vi "CIS.vi"(2 "Run uninterrupted?":bool, 3 "Device Category IN:":string(combo)="ATLAS18SS" caption="Device Category:", 4 "Structure:":string, 5 "Sensor Serial No.:":string, 6 "DB Serial No.:":string) -> (0 "Done!":bool)   [LabVIEW 2019]
doc: "Performs Cis measurements according to ATLAS ITk Quality Control Specifications."
uses:
  general_VIs/globals/QC_MeasurementSetup.vi
  general_VIs/globals/QC_RunInformation.vi
  InstrControl/InstrumentSetup.vi
  InstrControl/Switching/Switching.lvclass
  InstrControl/SupplyControl/SupplyControl.lvclass
  InstrControl/LCRControl/LCRControl.lvclass
  InstrControl/ArduinoControl/ArduinoControl.lvclass
  <vilib>/Analysis/NI_AALBase.lvlib
  InstrControl/InstrControl.lvclass
panel:
  out "Tab Control 2":enum32{"Cis Setup", "Cis Scan"}(tab)
  in  "Current Limit [µA]":dbl=1000.0 min=0.0001 format="%.3f"
  in  "Cis @300V limit [pF/cm]":dbl=1.0
  in  "step interval [s] IN":i32=5 caption="step interval [s]"
  in  "step [V] IN":dbl=10.0 caption="step [V]" format="%.1f"
  in  "Final volts [V] IN":dbl=-500.0 caption="Final volts [V]"
  in  "Initial volts [V] IN":dbl caption="Initial volts [V]"
  in  "Frequency [Hz] Setup":i32=500 caption="Frequency [Hz]" format="%#.3p"
  in  "Measurement Configurations":bool
  in  "Continue":bool
  in  "Quit":bool
  in  "Software current limit?":bool
  out "Capacitance":dbl[](array[numeric]) caption="Cap [pF]"
  out "Volts":dbl[](array[numeric]) caption="Volts [V]"
  out "Resistance":dbl[](array[numeric]) caption="Res [kOhm]"
  out "step interval [s]":u32=5
  out "step [V]":dbl=10.0 format="%.1f"
  out "Final volts [V]":dbl=-700.0 format="%.1f"
  out "Initial volts [V]":dbl format="%.1f"
  out "Frequency [Hz]":i32=100000 format="%#.3p"
  out "RH":dbl[](array[numeric]) caption="RH [%]" format="%#.2f"
  out "Temp.":dbl[](array[numeric]) caption="Temp. [°C]" format="%#.2f"
  out "Cgraph":cluster{"Initial volts":dbl, dbl, dbl[]}(graph)
  in  "Scales":T1(ring)
  in  "Cscale":enum16{"1/C^2 [1/nF^2]", "nF", "pF"}(ring)=enum."pF"
  out "positive ramp?":bool
  out "Tab Control":enum32{"Cis Setup", "Cis Scan"}(tab)
  in  "Switching":string(combo)="Pickering Matrix"
  in  "LCR Meter":string(combo)="WayneKerr 6440B"
  in  "Cis Supply":string(combo)="Keithley 2410"
  in  "Temperature":enum16{"Read Arduino", "Enter manually"}(ring)
  in  "User:":string(combo)="Christoph"
  in  "Manufacturer:":string(combo)="Hamamatsu"
  in  "abort":bool
  out "Device Category:":string
  out "DB Serial No.:":string
  out "Current Volts:":dbl format="%.2f"
  in  "quit (no save)":bool
  in  "Quit & Save":bool
  out "Bias On/Off:":bool
  out "STATUS 1":string
  out "Initiated:":string
  out "Sensor No.:":string
  out "No of steps":u32
  out "Current reading No.":u32
  out "Last reading at:":string
  # "University of\nCambridge"
  # "Strip Sensor QC: inter-strip Capacitance"
  # "Vertical Scale:"
  # "Measurement Configuration"
  # "Cis Scan parameters:"
  # "Last 5 readings:"
  # "n-4"
  # "n-3"
  # "n-2"
  # "n-1"
  # "n"
  # "DUT Description"
  # "Hardware"
  # "DUT & Test Description:"
  # "Current status:"
  # "Rdg No:"
  # "out of"
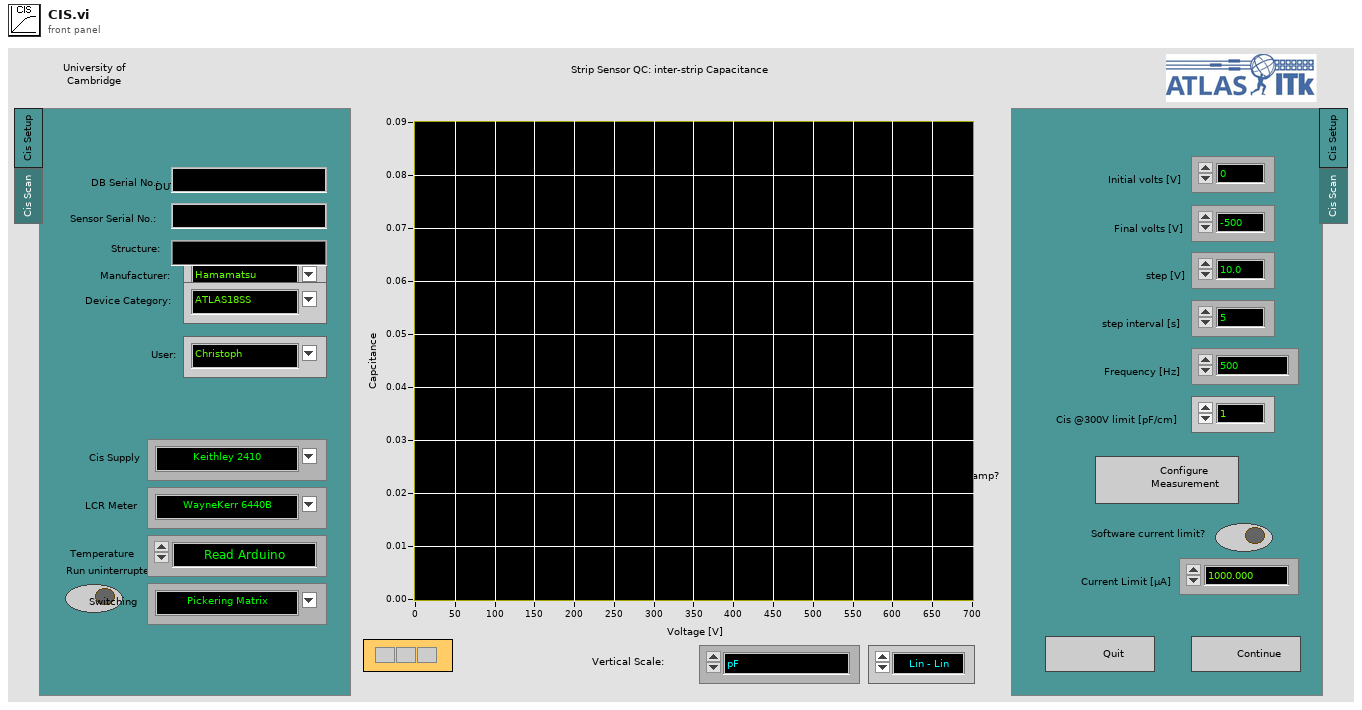
[diagram p1: front panel]
types:
  T1 = enum16{"Lin - Lin", "Log - Lin", "Lin - Log", "Log - log"}
  T2 = enum16{"Supply", "LCR", "Multimeter", "Switching"}
  T3 = enum16{"Reset", "Read Array", "Read Element", "Write Element", "Write Array", "Add Element", "Add Array"}
  T4 = enum16{"Reset", "Ground", "Striptest Bias", "Striptest SMU", "Striptest LCR", "IV", "CV", "Interstrip Cap", "Interstrip Res"}
  T5 = enum32{"IV", "CV", "Stability", "Striptest", "Cis", "Ris", "PTP"}
  T6 = cluster{"Sensor Serial No.:":string, "Wafer Serial No.:":string, "Batch:":string, "Manufacturer:":string, "Device Category:":string, "Database Serial No.:":string, "Date Initiated:":string, "Time Initiated:":string, "Test":string, "Instruments used:":string, "Probeplan used:":string, "End of Run comment:":string, "User:":string}
  T7 = cluster{"Institute":string, "Manufacturers":string[], "Devices":string[], "Serialnumbers Lookup DB":string, "Data directory":string, "Backup & screenshot directory":string, "List of known users":string[], "Measurement switch not used":bool, "Measurement Switch":string, "DUT Switch":string}
  T8 = cluster{"Supply":refnum<class "SupplyControl.lvclass">, "LCR":refnum<class "LCRControl.lvclass">, "Initial Voltage [V]":dbl, "Final Voltage [V]":dbl, "Step Size [V]":dbl, "Step Interval [s]":i32, "Number Of Steps":u32, "AC frequency [Hz]":i32, "RC Configuration":u16, "AC amplitude [V]":dbl, "Ramp down steps [V]":dbl, "Ramp down Interval [s]":i32, "Set Current Limit?":bool, "Current Limit [µA]":dbl, "Temperature Readout":enum16{"Read Arduino", "Enter manually"}, "Arduino":refnum<class "ArduinoControl.lvclass">, "Supply Name":string, "LCR Name":string, "C_is Limit [pF/cm]":dbl, "Switching":refnum<class "Switching.lvclass">, "Matrix used?":bool, "Matrix X Channels":cluster{"Bias Supply / SMU LO":i32, "Bias Supply / SMU HI":i32, "CV Box LO":i32, "CV Box HI":i32, "CV Box LO IN":i32, "CV Box HI IN":i32, "Volt meter LO":i32, "Volt meter HI":i32, "Mux1 C1":i32, "Mux1 C2":i32, "Mux2 C1":i32, "Mux2 C2":i32}, "Structure Name":string}
  T9 = cluster{"VISA address":refnum<visa-resource-name>, "T sensor":enum16{"SHT", "DS"}, "Arduino":refnum<class "ArduinoControl.lvclass">}
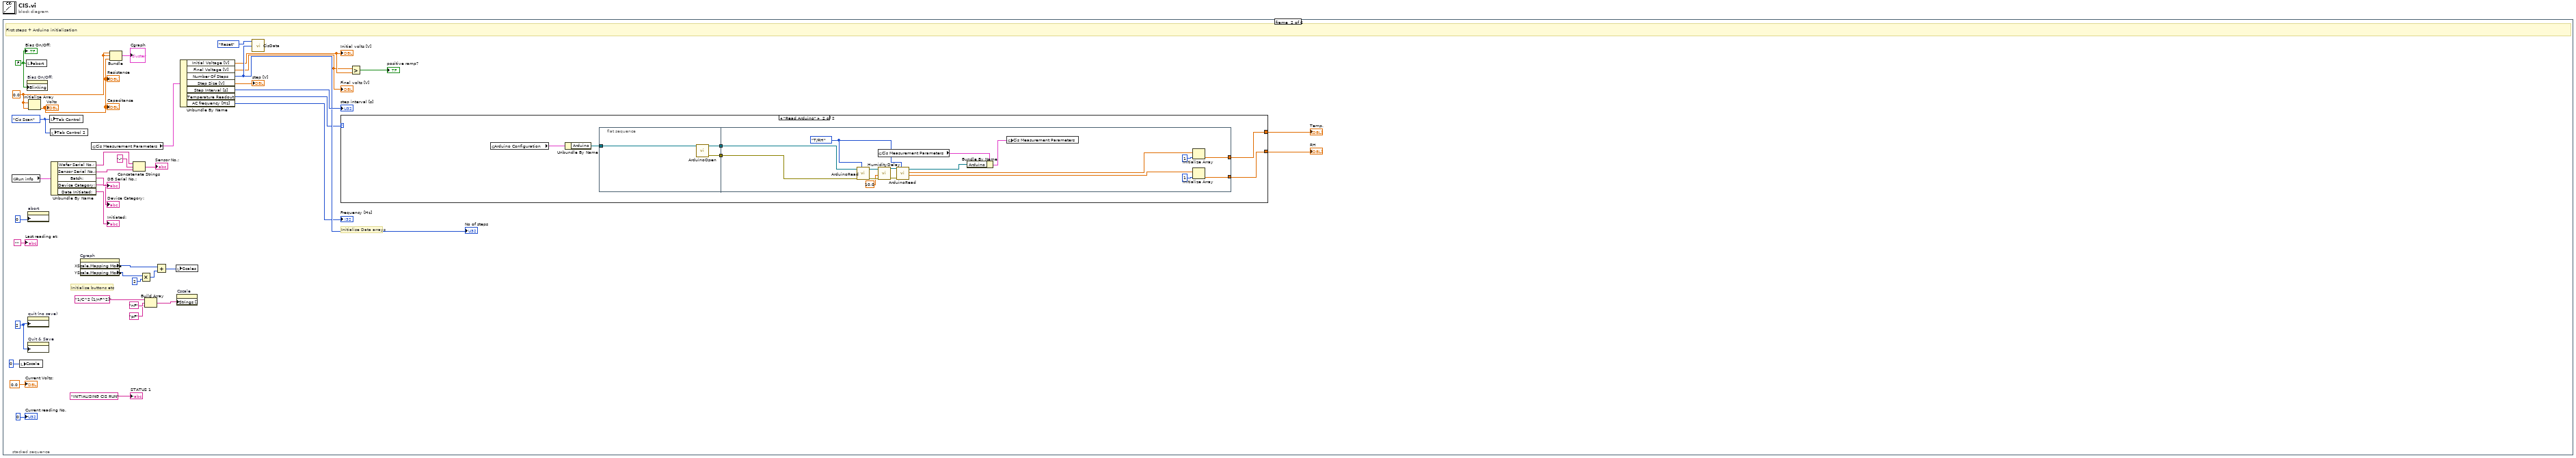
[diagram p0: block diagram]
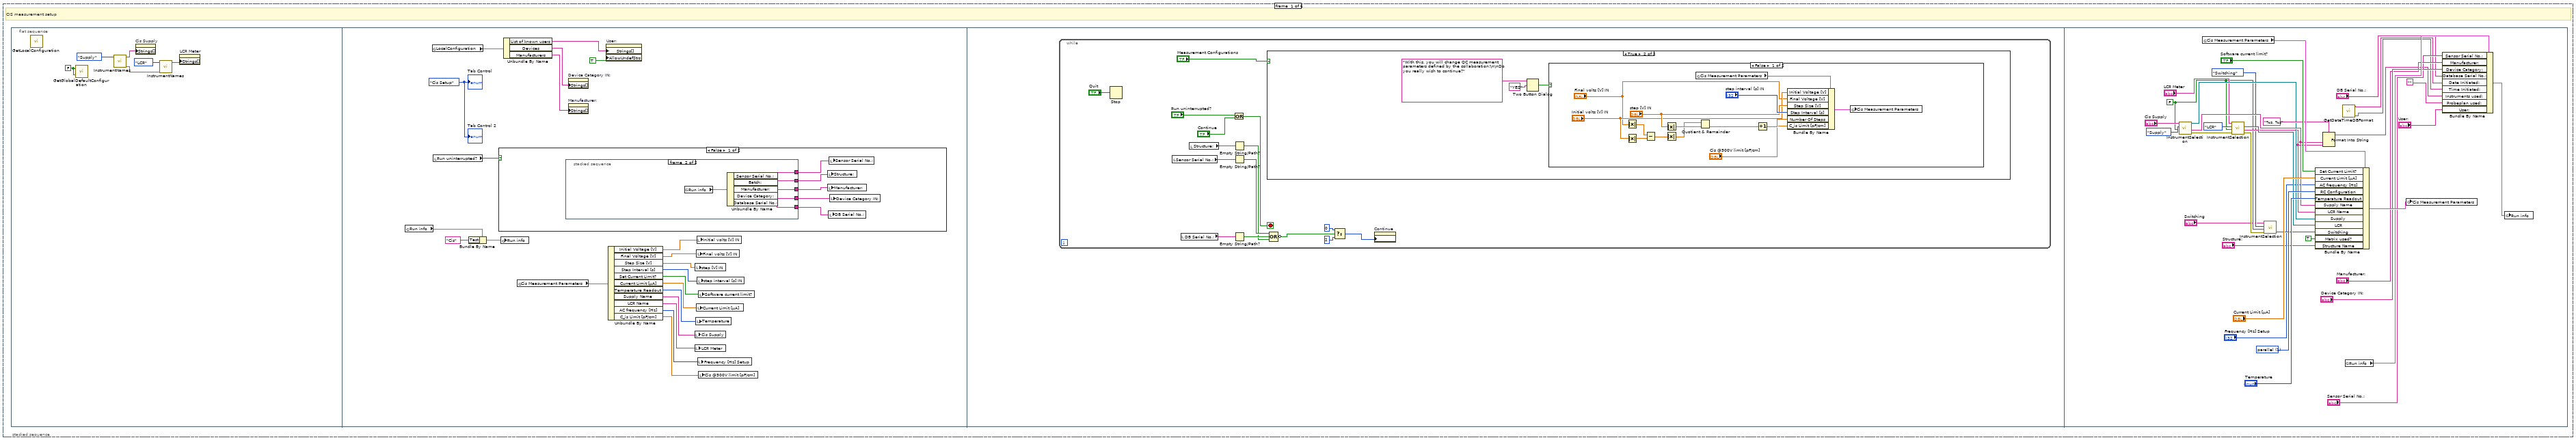
[diagram p2: hidden frame]
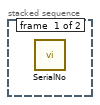
[diagram p3: hidden frame]
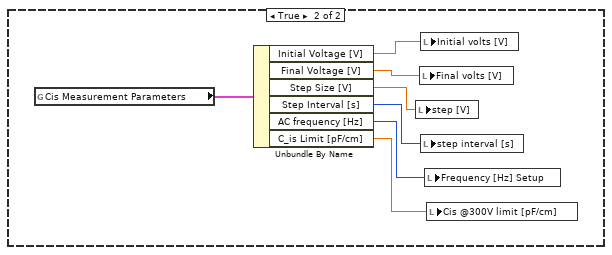
[diagram p6: hidden frame]
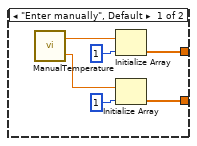
[diagram p7: hidden frame]
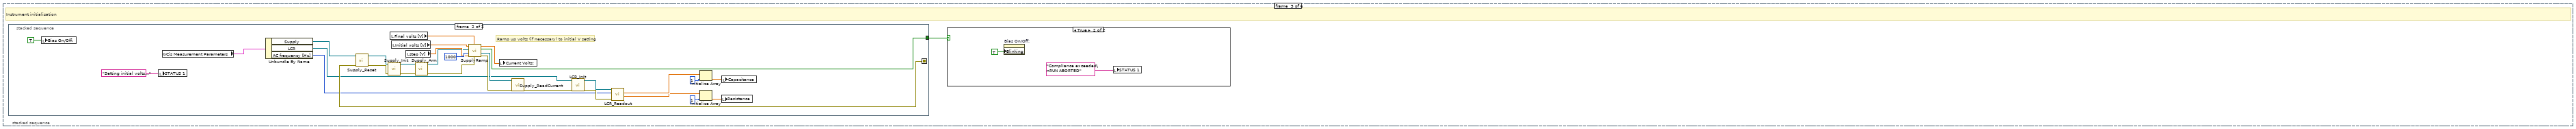
[diagram p8: hidden frame]
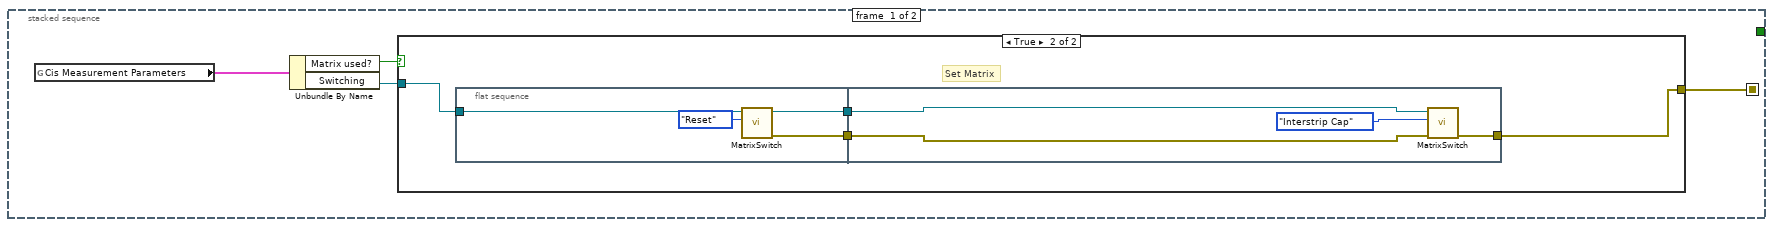
[diagram p9: hidden frame]
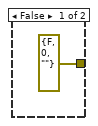
[diagram p10: hidden frame]
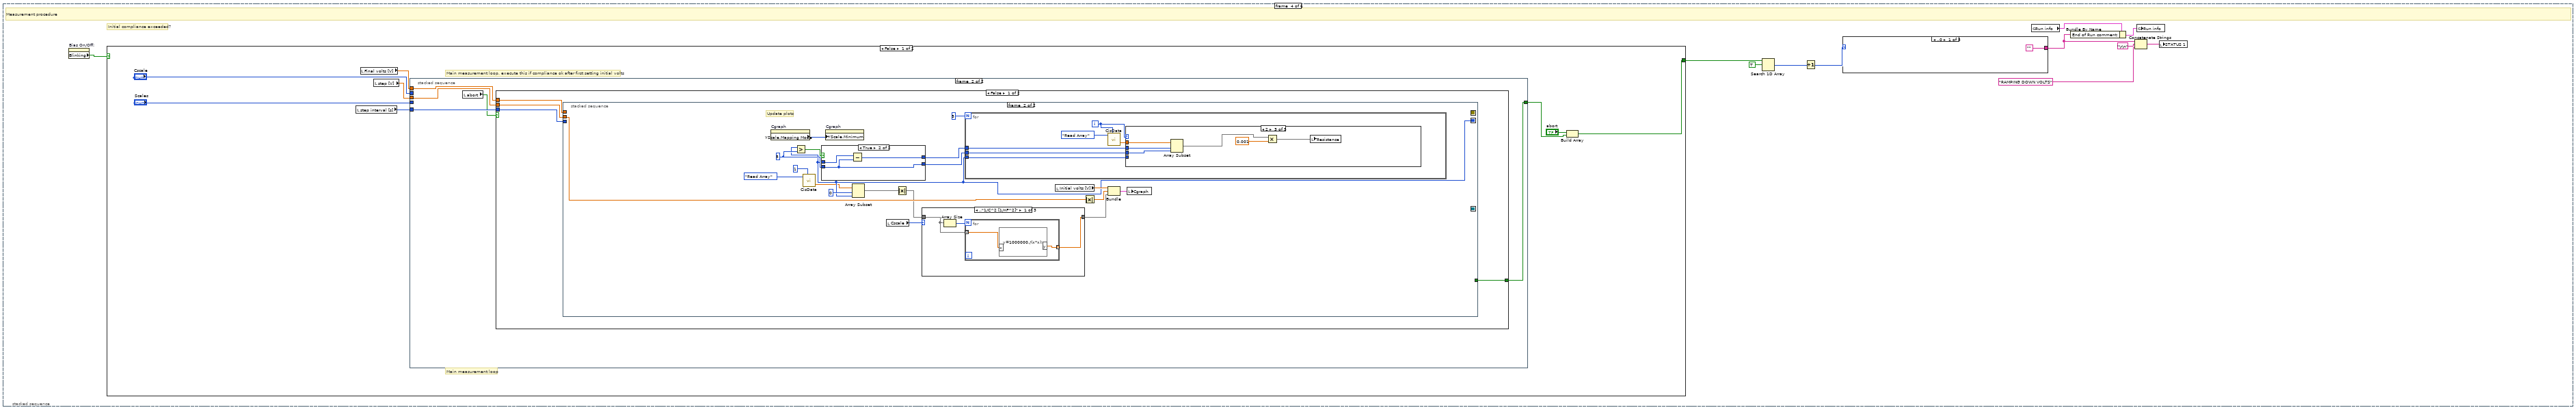
[diagram p12: hidden frame]
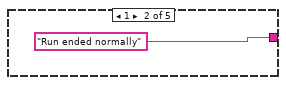
[diagram p13: hidden frame]
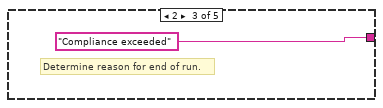
[diagram p14: hidden frame]
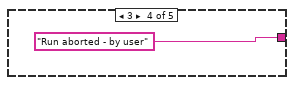
[diagram p15: hidden frame]
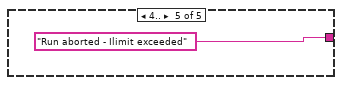
[diagram p16: hidden frame]
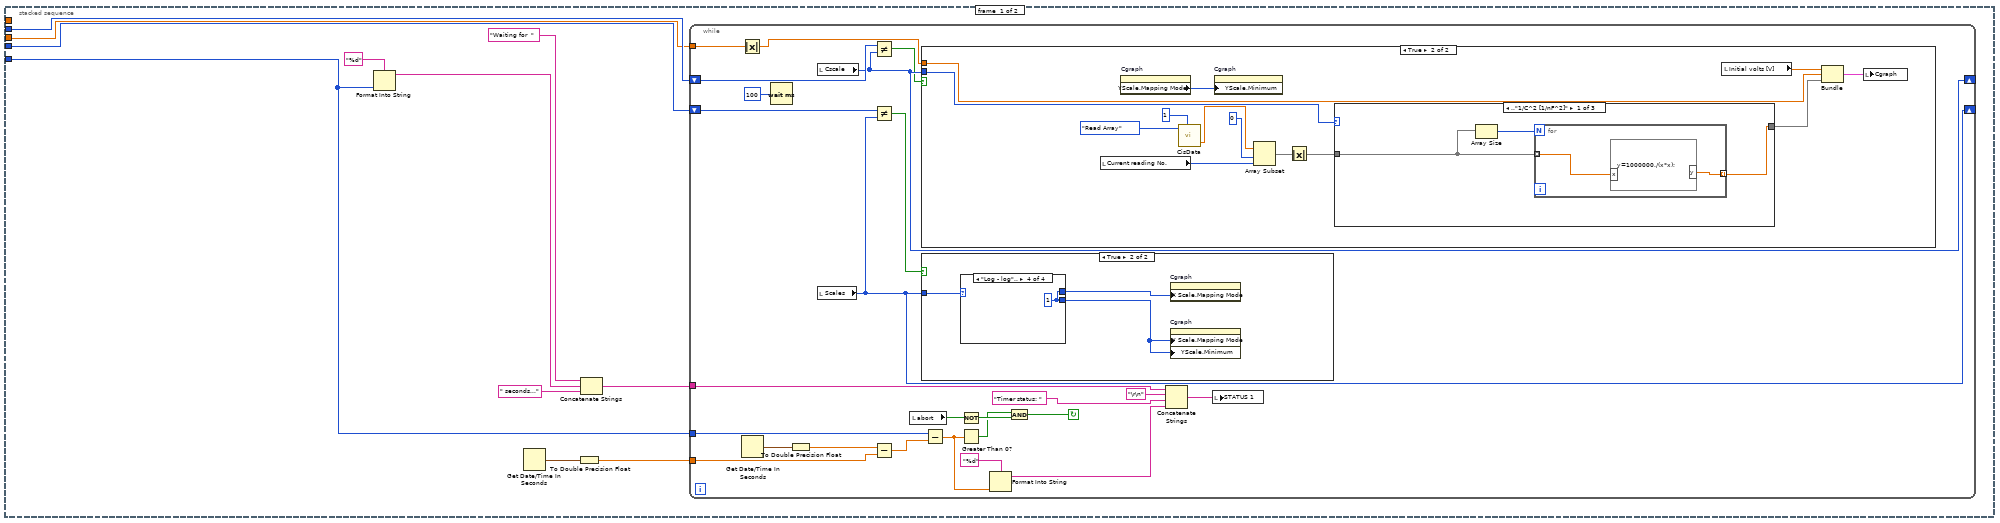
[diagram p17: hidden frame]
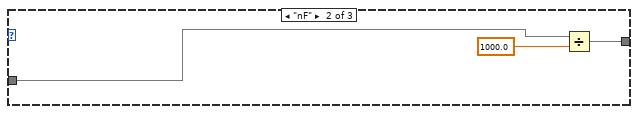
[diagram p19: hidden frame]
diagram:
  n1 = stacked-sequence {
    frame #0 {
      # "CIS measurement setup"
      n2 = flat-sequence {
        frame #0 {
          w6 = FALSE
          n3 = call "GetLocalConfiguration.vi"() -> ()  [unwired: 3 in, 1 out]
          n4 = call "GetGlobalDefaultConfiguration.vi"("DO NOT override instruments"=w6, "Read defaults?"=w6) -> ()  [unwired: 1 in, 1 out]
          n5 = call "InstrumentNames.vi"("Instrument type"=T2."Supply") -> ("error out"=w3:errorcluster, "Instrument names"=w1:string[])  [unwired: 9 in]
          n6 = property on="Cis Supply" class="CmbBox"("Strings[]"=w1) -> ()  [unwired: 2 in, 2 out]
          n7 = call "InstrumentNames.vi"("error in (no error)"=w3, "Instrument type"=T2."LCR") -> ("Instrument names"=w2:string[])  [unwired: 8 in, 1 out]
          n8 = property on="LCR Meter" class="CmbBox"("Strings[]"=w2) -> ()  [unwired: 2 in, 2 out]
        }
        frame #1 {
          w15 = enum32{"Cis Setup", "Cis Scan"}."Cis Setup" ("Tab Control")
          n9 = global read "QC_RunInformation.vi" "Run info"() -> (w16:T6)
          n10 = global read "QC_RunInformation.vi" "LocalConfiguration"() -> (w23:T7)
          n11 = local read "Run uninterrupted?"() -> (w14:bool)
          n12 = Bundle By Name(cluster=w16, "Test"="Cis") -> (w18:T6)
          n13 = case shown="False" w14 {
            frame False {
              n14 = stacked-sequence {
                tunnel: [_ w39] -> w33
                tunnel: [_ w38] -> w32
                tunnel: [_ w37] -> w31
                tunnel: [_ w36] -> w29
                tunnel: [_ w34] -> w30
                frame #0 {
                  n15 = call "SerialNo.vi"() -> ()  [unwired: 5 in, 1 out]
                }
                frame #1 {
                  n16 = global read "QC_RunInformation.vi" "Run info"() -> (w35:T6)
                  n17 = Unbundle By Name(w35) -> ("Sensor Serial No.:"=w39:string, "Batch:"=w38:string, "Manufacturer:"=w37:string, "Device Category:"=w36:string, "Database Serial No.:"=w34:string)
                }
              }
              n18 = local write "Structure:"(w32) -> ()
              n19 = local write "Manufacturer:"(w31) -> ()
              n20 = local write "DB Serial No.:"(w30) -> ()
              n21 = local write "Sensor Serial No.:"(w33) -> ()
              n22 = local write "Device Category IN:"(w29) -> ()
            }
            frame True {
            }
          }
          n23 = global write "QC_RunInformation.vi" "Run info"(w18) -> ()
          n24 = Unbundle By Name(w23) -> ("List of known users"=w22:string[], "Devices"=w7:string[], "Manufacturers"=w8:string[])
          n25 = global read "QC_MeasurementSetup.vi" "Cis Measurement Parameters"() -> (w26:T8)
          n26 = property on="Device Category IN:" class="CmbBox"("Strings[]"=w7) -> ()  [unwired: 2 in, 2 out]
          n27 = property on="Manufacturer:" class="CmbBox"("Strings[]"=w8) -> ()  [unwired: 2 in, 2 out]
          n28 = property on="User:" class="CmbBox"("Strings[]"=w22, "AllowUndefStrs"=TRUE) -> ()  [unwired: 2 in, 2 out]
          n29 = Unbundle By Name(w26) -> ("Initial Voltage [V]"=w11:dbl, "Final Voltage [V]"=w12:dbl, "Step Size [V]"=w10:dbl, "Step Interval [s]"=w13:i32, "Set Current Limit?"=w25:bool, "Current Limit [µA]"=w24:dbl, "Temperature Readout"=w28:enum16{"Read Arduino", "Enter manually"}, "Supply Name"=w27:string, "LCR Name"=w20:string, "AC frequency [Hz]"=w19:i32, "C_is Limit [pF/cm]"=w9:dbl)
          n30 = local write "Cis Supply"(w27) -> ()
          n31 = local write "LCR Meter"(w20) -> ()
          n32 = local write "step [V] IN"(w10) -> ()
          n33 = local write "Temperature"(w28) -> ()
          n34 = local write "Final volts [V] IN"(w12) -> ()
          n35 = local write "Current Limit [µA]"(w24) -> ()
          n36 = local write "Initial volts [V] IN"(w11) -> ()
          n37 = local write "step interval [s] IN"(w13) -> ()
          n38 = local write "Frequency [Hz] Setup"(w19) -> ()
          n39 = local write "Software current limit?"(w25) -> ()
          n40 = local write "Cis @300V limit [pF/cm]"(w9) -> ()
          "Tab Control" <- w15
          "Tab Control 2" <- w15
        }
        frame #2 {
          n41 = while {
            stop <- w41 stop-if-true
            n42 = Stop(stop? (T)="Quit") -> ()
            n43 = local read "Sensor Serial No.:"() -> (w53:string)
            n44 = local read "DB Serial No.:"() -> (w52:string)
            n45 = local read "Structure:"() -> (w45:string)
            n46 = Or(x="Run uninterrupted?", y="Continue") -> (x .or. y?=w41:bool)
            n47 = Empty String/Path?(string/path=w45) -> (empty?=w44:bool)
            n48 = Empty String/Path?(string/path=w53) -> (empty?=w50:bool)
            n49 = Empty String/Path?(string/path=w52) -> (empty?=w51:bool)
            n50 = case shown="True" "Measurement Configurations" {
              frame False {
              }
              frame True {
                n51 = Two Button Dialog(message="With this, you will change QC measurement parameters defined by the collaboration!\n\nDo you really wish to continue?", 2:"YES") -> (T button?=w55:bool)  [unwired: 1 in]
                n52 = case shown="False" w55 {
                  frame False {
                    n53 = Absolute Value(x="Final volts [V] IN") -> (abs(x)=w68:dbl)
                    n54 = Absolute Value(x="Initial volts [V] IN") -> (abs(x)=w67:dbl)
                    n55 = Subtract(x=w68, y=w67) -> (x-y=w65:dbl)
                    n56 = Absolute Value(x="step [V] IN") -> (abs(x)=w66:dbl)
                    n57 = Absolute Value(x=w65) -> (abs(x)=w61:dbl)
                    n58 = global read "QC_MeasurementSetup.vi" "Cis Measurement Parameters"() -> (w70:T8)
                    n59 = Quotient & Remainder(x=w61, y=w66) -> (floor(x/y)=w69:dbl)  [unwired: 1 out]
                    n60 = Increment(x=w69) -> (x+1=w64:dbl)
                    n61 = Bundle By Name(cluster=w70, "Initial Voltage [V]"="Initial volts [V] IN", "Final Voltage [V]"="Final volts [V] IN", "Step Size [V]"="step [V] IN", "Step Interval [s]"="step interval [s] IN", "Number Of Steps"=w64, "C_is Limit [pF/cm]"="Cis @300V limit [pF/cm]") -> (w71:T8)
                    n62 = global write "QC_MeasurementSetup.vi" "Cis Measurement Parameters"(w71) -> ()
                  }
                  frame True {
                    n63 = global read "QC_MeasurementSetup.vi" "Cis Measurement Parameters"() -> (w78:T8)
                    n64 = Unbundle By Name(w78) -> ("Initial Voltage [V]"=w76:dbl, "Final Voltage [V]"=w77:dbl, "Step Size [V]"=w75:dbl, "Step Interval [s]"=w74:i32, "AC frequency [Hz]"=w73:i32, "C_is Limit [pF/cm]"=w72:dbl)
                    n65 = local write "step [V]"(w75) -> ()
                    n66 = local write "Final volts [V]"(w77) -> ()
                    n67 = local write "Initial volts [V]"(w76) -> ()
                    n68 = local write "step interval [s]"(w74) -> ()
                    n69 = local write "Frequency [Hz] Setup"(w73) -> ()
                    n70 = local write "Cis @300V limit [pF/cm]"(w72) -> ()
                  }
                }
              }
            }
            n71 = Compound Arithmetic op=OR(w50, w51, w44) -> (invert w49:bool)
            n72 = Select(t=0, s=w49, f=2) -> (s? t:f=w46:i32)
            n73 = property on="Continue" class="Bool"("DisabledEnum"=w46) -> ()  [unwired: 2 in, 2 out]
          }
        }
        frame #3 {
          w87 = FALSE
          w102 = u16 1 items=["serial", "parallel"] ("RC Configuration")
          n74 = call "InstrumentSelection.vi"("Verify GPIB address"=w87, "Instrument type"=T2."Supply", "Instrument name IN"="Cis Supply") -> ("error out"=w92:errorcluster, "Instrument name OUT"=w97:string, "Supply"=w96:refnum<class "SupplyControl.lvclass">)  [unwired: 3 in, 3 out]
          n75 = global read "QC_MeasurementSetup.vi" "Cis Measurement Parameters"() -> (w112:T8)
          n76 = call "InstrumentSelection.vi"("error in (no error)"=w92, "Verify GPIB address"=w87, "Instrument type"=T2."LCR", "Instrument name IN"="LCR Meter") -> ("error out"=w88:errorcluster, "Instrument name OUT"=w93:string, "LCR"=w95:refnum<class "LCRControl.lvclass">)  [unwired: 2 in, 3 out]
          n77 = call "InstrumentSelection.vi"("error in (no error)"=w88, "Verify GPIB address"=w87, "Instrument type"=T2."Switching", "Instrument name IN"="Switching") -> ("Switching"=w86:refnum<class "Switching.lvclass">)  [unwired: 2 in, 5 out]
          n78 = Bundle By Name(cluster=w112, "Set Current Limit?"="Software current limit?", "Current Limit [µA]"="Current Limit [µA]", "AC frequency [Hz]"="Frequency [Hz] Setup", "RC Configuration"=w102, "Temperature Readout"="Temperature", "Supply Name"=w97, "LCR Name"=w93, "Supply"=w96, "LCR"=w95, "Switching"=w86, "Matrix used?"=TRUE, "Structure Name"="Structure:") -> (w113:T8)
          n79 = Format Into String(format string="%s, %s", w97, w93) -> (resulting string=w99:string)  [unwired: 2 in, 1 out]
          n80 = call "GetDateTimeDBFormat.vi"() -> ("Time in 24h format, e.g. 13:40:54"=w79:string, "Abbreviated Date, e.g. 13 Nov 2020"=w80:string)  [unwired: 10 in]
          n81 = global read "QC_RunInformation.vi" "Run info"() -> (w109:T6)
          n82 = global write "QC_MeasurementSetup.vi" "Cis Measurement Parameters"(w113) -> ()
          n83 = Bundle By Name(cluster=w109, "Sensor Serial No.:"="Sensor Serial No.:", "Manufacturer:"="Manufacturer:", "Device Category:"="Device Category IN:", "Database Serial No.:"="DB Serial No.:", "Date Initiated:"=w80, "Time Initiated:"=w79, "Instruments used:"=w99, "Probeplan used:"="", "User:"="User:") -> (w108:T6)
          n84 = global write "QC_RunInformation.vi" "Run info"(w108) -> ()
        }
      }
    }
    frame #1 {
      w114 = enum32{"Cis Setup", "Cis Scan"}."Cis Scan" ("Tab Control")
      w136 = 2
      w143 = 0.0
      w135 = FALSE ("Visible")
      # "Initialise buttons etc"
      # "Initialise Data arrays"
      # "First steps + Arduino initialisation"
      n85 = global read "QC_RunInformation.vi" "Run info"() -> (w153:T6)
      n86 = local write "Cscale"(u16 0 ("Scale")) -> ()
      n87 = local write "abort"(w135) -> ()
      n88 = property on="Bias On/Off:" class="Bool (strict)"("Blinking"=w135) -> ()  [unwired: 2 in, 2 out]
      n89 = property on="abort" class="Bool (strict)"("DisabledEnum"=0) -> ()  [unwired: 2 in, 2 out]
      n90 = property on="quit (no save)" class="Bool"("DisabledEnum"=w136) -> ()  [unwired: 2 in, 2 out]
      n91 = property on="Quit & Save" class="Bool"("DisabledEnum"=w136) -> ()  [unwired: 2 in, 2 out]
      n92 = Initialize Array(w143, w143) -> (w116:dbl[])
      "Volts" <- w116
      "Capacitance" <- w116
      "Resistance" <- w116
      n93 = local write "Tab Control"(w114) -> ()
      n94 = local write "Tab Control 2"(w114) -> ()
      n95 = Unbundle By Name(w153) -> ("Wafer Serial No.:"=w122:string, "Sensor Serial No.:"=w121:string, "Batch:"=→"DB Serial No.:":string, "Device Category:"=→"Device Category:":string, "Date Initiated:"=→"Initiated:":string)
      n96 = property on="Cgraph" class="WFGraph (strict)"() -> ("XScale.Mapping Mode"=w128:u8, "YScale.Mapping Mode"=w127:u8)  [unwired: 2 in, 2 out]
      n97 = global read "QC_MeasurementSetup.vi" "Cis Measurement Parameters"() -> (w124:T8)
      n98 = Bundle(w143, w143, w116) -> (→"Cgraph":cluster{dbl, dbl, dbl[]})  [unwired: 1 in]
      n99 = Concatenate Strings(w122, "-", w121) -> (→"Sensor No.:":string)
      n100 = Multiply(x=w127, y=2) -> (x*y=w130:i32)
      n101 = Build Array("1/C^2 [1/nF^2]", "nF", "pF") -> (w150:string[])
      n102 = Add(x=w128, y=w130) -> (x+y=w126:i32)
      n103 = local write "Scales"(w126) -> ()
      n104 = property on="Cscale" class="Enum (strict)"("Strings []"=w150) -> ()  [unwired: 2 in, 2 out]
      n105 = Unbundle By Name(w124) -> ("Initial Voltage [V]"=w134:dbl, "Final Voltage [V]"=w133:dbl, "Number Of Steps"=w144:u32, "Step Size [V]"=→"step [V]":dbl, "Step Interval [s]"=→"step interval [s]":i32, "Temperature Readout"=w137:enum16{"Read Arduino", "Enter manually"}, "AC frequency [Hz]"=→"Frequency [Hz]":i32)
      "No of steps" <- w144
      "Initial volts [V]" <- w134
      "Final volts [V]" <- w133
      n106 = call "CisData.vi"("Action"=T3."Reset", "Array Size / Index"=w144) -> ()  [unwired: 3 in, 2 out]
      n107 = case shown="\"Read Arduino\"" w137 {
        tunnel: [w159 w166] -> w140
        tunnel: [w156 w165] -> w125
        frame "Enter manually", Default {
          n108 = call "ManualTemperature.vi"() -> ("Humidity [%] out"=w155:dbl, "Temperature [°C] out"=w160:dbl)
          n109 = Initialize Array(w160, 1) -> (w159:dbl[])
          n110 = Initialize Array(w155, 1) -> (w156:dbl[])
        }
        frame "Read Arduino" {
          n111 = global read "InstrumentSetup.vi" "Arduino Configuration"() -> (w162:T9)
          n112 = Unbundle By Name(w162) -> ("Arduino"=w161:refnum<class "ArduinoControl.lvclass">)
          n113 = flat-sequence {
            tunnel: [w167] -> w164
            tunnel: [w169] -> w163
            tunnel: w161 -> [w168]
            tunnel: [w186] -> w166
            tunnel: [w183] -> w165
            tunnel: w164 -> [w175]
            tunnel: w163 -> [w176]
            frame #0 {
              n114 = call "ArduinoOpen.vi"("ArduinoControl in"=w168) -> ("error out"=w169:errorcluster, "ArduinoControl out"=w167:refnum<class "ArduinoControl.lvclass">)  [unwired: 9 in]
            }
            frame #1 {
              w177 = enum16{"T/RH", "Interlock", "Edgesense"}."T/RH" ("Arduino function")
              n115 = call "ArduinoRead.vi"("Arduino function"=w177, "error in (no error)"=w176, "ArduinoControl in"=w175) -> ("error out"=w174:errorcluster, "ArduinoControl out"=w173:refnum<class "ArduinoControl.lvclass">)  [unwired: 3 in, 4 out]
              n116 = global read "QC_MeasurementSetup.vi" "Cis Measurement Parameters"() -> (w179:T8)
              n117 = call "HumidityDelay.vi"("error in (no error)"=w174, "Start Humidity"=10.0, "ArduinoControl in"=w173) -> ("error out"=w171:errorcluster, "ArduinoControl out"=w172:refnum<class "ArduinoControl.lvclass">)  [unwired: 7 in]
              n118 = call "ArduinoRead.vi"("Arduino function"=w177, "error in (no error)"=w171, "ArduinoControl in"=w172) -> ("rel. Humidity [%]"=w181:dbl, "Temperature [°C]"=w182:dbl, "ArduinoControl out"=w180:refnum<class "ArduinoControl.lvclass">)  [unwired: 3 in, 3 out]
              n119 = Bundle By Name(cluster=w179, "Arduino"=w180) -> (w178:T8)
              n120 = global write "QC_MeasurementSetup.vi" "Cis Measurement Parameters"(w178) -> ()
              n121 = Initialize Array(w182, 1) -> (w186:dbl[])
              n122 = Initialize Array(w181, 1) -> (w183:dbl[])
            }
          }
        }
      }
      "Temp." <- w140
      "RH" <- w125
      n123 = Greater?(x=w133, y=w134) -> (0:→"positive ramp?":bool)
      "STATUS 1" <- "INITIALISING CIS RUN"
      "Bias On/Off:" <- w135
      "Last reading at:" <- ""
      "Current reading No." <- u32 0 ("Current reading No.")
      "Current Volts:" <- 0.0 ("Current Volts:")
    }
    frame #2 {
      # "Instrument initialisation"
      n124 = stacked-sequence {
        seq-local: [w189 _] -> [_ w210]
        tunnel: [_ w211] -> w187
        frame #0 {
          n125 = global read "QC_MeasurementSetup.vi" "Cis Measurement Parameters"() -> (w188:T8)
          n126 = Unbundle By Name(w188) -> ("Matrix used?"=w191:bool, "Switching"=w190:refnum<class "Switching.lvclass">)
          n127 = case shown="True" w191 {
            tunnel: w190 -> [_ w193]
            tunnel: [errorcluster {"status"=FALSE, "code"=0, "source"=""} ("error constant") w194] -> w189
            frame False {
            }
            frame True {
              # "Set Matrix"
              n128 = flat-sequence {
                tunnel: [w200] -> w196
                tunnel: [w199] -> w195
                tunnel: w193 -> [w198]
                tunnel: w196 -> [w204]
                tunnel: w195 -> [w203]
                tunnel: [w202] -> w194
                frame #0 {
                  n129 = call-dynamic "MatrixSwitch.vi"("Action"=T4."Reset", "Switching in"=w198) -> ("error out"=w200:errorcluster, "Switching out"=w199:refnum<class "Switching.lvclass">)  [unwired: 7 in, 1 out]
                }
                frame #1 {
                  n130 = call-dynamic "MatrixSwitch.vi"("error in (no error)"=w204, "Action"=T4."Interstrip Cap", "Switching in"=w203) -> ("error out"=w202:errorcluster)  [unwired: 6 in, 2 out]
                }
              }
            }
          }
        }
        frame #1 {
          # "Ramp up volts (if necessary) to initial V setting"
          n131 = local write "Bias On/Off:"(TRUE ("Compliance?")) -> ()
          n132 = local write "STATUS 1"("Setting initial volts..." ("STATUS 1")) -> ()
          n133 = global read "QC_MeasurementSetup.vi" "Cis Measurement Parameters"() -> (w230:T8)
          n134 = Unbundle By Name(w230) -> ("Supply"=w227:refnum<class "SupplyControl.lvclass">, "LCR"=w208:refnum<class "LCRControl.lvclass">, "AC frequency [Hz]"=w207:i32)
          n135 = call-dynamic "Supply_Reset.vi"("error in (no error)"=w210, "SupplyControl in"=w227) -> ("error out"=w232:errorcluster, "SupplyControl out"=w234:refnum<class "SupplyControl.lvclass">)  [unwired: 8 in]
          n136 = call-dynamic "Supply_Init.vi"("error in (no error)"=w232, "SupplyControl in"=w234) -> ("error out"=w231:errorcluster, "SupplyControl out"=w233:refnum<class "SupplyControl.lvclass">)  [unwired: 8 in]
          n137 = local read "Final volts [V]"() -> (w205:dbl)
          n138 = local read "Initial volts [V]"() -> (w206:dbl)
          n139 = local read "step [V]"() -> (w214:dbl)
          n140 = call-dynamic "Supply_Arm.vi"("error in (no error)"=w231, "SupplyControl in"=w233) -> ("error out"=w212:errorcluster, "SupplyControl out"=w213:refnum<class "SupplyControl.lvclass">)  [unwired: 8 in]
          n141 = call "SupplyRamp.vi"("error in"=w212, "Requested Voltage"=w205, "Step Size"=w214, "Step Delay"=1000, "Supply IN"=w213, "Starting Voltage"=w206) -> ("error out"=w226:errorcluster, "Supply OUT"=w209:refnum<class "SupplyControl.lvclass">, "Compliance exceeded"=w211:bool, "Current Voltage"=w216:dbl)  [unwired: 2 in]
          n142 = local write "Current Volts:"(w216) -> ()
          n143 = call-dynamic "Supply_ReadCurrent.vi"("error in (no error)"=w226, "SupplyControl in"=w209) -> ("error out"=w223:errorcluster)  [unwired: 7 in, 2 out]
          n144 = call-dynamic "LCR_Init.vi"("error in (no error)"=w223, "LCRControl in"=w208) -> ("error out"=w225:errorcluster, "LCRControl out"=w224:refnum<class "LCRControl.lvclass">)  [unwired: 8 in]
          n145 = call-dynamic "LCR_Readout.vi"("error in (no error)"=w225, "Frequency in Hz"=w207, "LCRControl in"=w224) -> ("Resistance in Ohm"=w221:dbl, "Capacitance in pF"=w222:dbl)  [unwired: 5 in, 2 out]
          n146 = Initialize Array(w222, 1) -> (w217:dbl[])
          n147 = Initialize Array(w221, 1) -> (w220:dbl[])
          n148 = local write "Resistance"(w220) -> ()
          n149 = local write "Capacitance"(w217) -> ()
        }
      }
      n150 = case shown="True" w187 {
        frame False {
        }
        frame True {
          n151 = property on="Bias On/Off:" class="Bool (strict)"("Blinking"=TRUE) -> ()  [unwired: 2 in, 2 out]
          n152 = local write "STATUS 1"("Compliance exceeded\nRUN ABORTED") -> ()
        }
      }
    }
    frame #3 {
      # "Initial compliance exceeded?"
      # "Measurement procedure"
      n153 = property on="Bias On/Off:" class="Bool (strict)"() -> ("Blinking"=w247:bool)  [unwired: 2 in, 2 out]
      n154 = case shown="False" w247 {
        tunnel: [w260 w448] -> w246
        frame False {
          # "Main measurement loop"
          # "Main measurement loop. execute this if compliance ok after first setting initial volts"
          n155 = local read "step interval [s]"() -> (w255:u32)
          n156 = local read "Final volts [V]"() -> (w256:dbl)
          n157 = local read "step [V]"() -> (w257:dbl)
          n158 = stacked-sequence {
            tunnel: w257 -> [w269 w332]
            tunnel: w256 -> [_ w331]
            tunnel: w255 -> [w261 w330]
            tunnel: "Scales" -> [w271 _]
            tunnel: "Cscale" -> [w270 _]
            tunnel: [_ w328] -> w254
            frame #0 {
              n159 = Format Into String(format string="%d", w261) -> (resulting string=w266:string)  [unwired: 2 in, 1 out]
              n160 = Get Date/Time In Seconds() -> (seconds since 1Jan1904=w263:timestamp)
              n161 = To Double Precision Float(number=w263) -> (double precision float=w264:dbl)
              n162 = Concatenate Strings("Waiting for  ", w266, " seconds...") -> (w262:string)
              n163 = while {
                tunnel: w269 -> [w280]
                shift-left: w270 -> [w284]
                shift-right: [w277] -> _
                shift-left: w271 -> [w285]
                shift-right: [w286] -> _
                tunnel: w262 -> [w278]
                tunnel: w261 -> [w290]
                tunnel: w264 -> [w291]
                stop <- w292 continue-if-true
                n164 = Absolute Value(x=w280) -> (abs(x)=w279:dbl)
                n165 = Get Date/Time In Seconds() -> (seconds since 1Jan1904=w276:timestamp)
                n166 = Wait (ms)(milliseconds to wait=u32 100) -> ()  [unwired: 1 out]
                n167 = To Double Precision Float(number=w276) -> (double precision float=w296:dbl)
                n168 = local read "Cscale"() -> (w277:enum16{"1/C^2 [1/nF^2]", "nF", "pF"})
                n169 = local read "Scales"() -> (w286:T1)
                n170 = Not Equal?(x=w284, y=w277) -> (x != y?=w275:bool)
                n171 = Not Equal?(x=w285, y=w286) -> (x != y?=w287:bool)
                n172 = Subtract(x=w296, y=w291) -> (x-y=w273:dbl)
                n173 = local read "abort"() -> (w289:bool)
                n174 = case shown="True" w275 {
                  tunnel: w279 -> [_ w308]
                  tunnel: w277 -> [_ w301]
                  frame False {
                  }
                  frame True {
                    n175 = local read "Current reading No."() -> (w306:u32)
                    n176 = property on="Cgraph" class="WFGraph (strict)"() -> ("YScale.Mapping Mode"=w303:u8)  [unwired: 2 in, 2 out]
                    n177 = call "CisData.vi"("Action"=T3."Read Array", "Array No."=u32 1 ("Action")) -> ("Array OUT"=w297:dbl[])  [unwired: 3 in, 1 out]
                    n178 = property on="Cgraph" class="WFGraph (strict)"("YScale.Minimum"=w303) -> ()  [unwired: 2 in, 2 out]
                    n179 = Array Subset(array=w297, index=0, length=w306) -> (w304:dbl[])
                    n180 = Absolute Value(x=w304) -> (abs(x)=w302:dbl[])
                    n181 = case shown="..\"1/C^2 [1/nF^2]\"" w301 {
                      tunnel: [w312 w315 w318] -> w300
                      tunnel: w302 -> [w310 w317 w318]
                      frame .."1/C^2 [1/nF^2]" {
                        n182 = Array Size(array=w310) -> (size(s)=w311:i32)
                        n183 = for {
                          N: w311 -> [_]
                          tunnel: w310 -> [w314] mode=indexing
                          tunnel: [w313] -> w312 mode=indexing
                          n184 = formula code="y=1000000./(x*x);"("x"=w314) -> ("y"=w313:dbl)
                        }
                      }
                      frame "nF" {
                        n185 = Divide(x=w317, y=1000.0) -> (x/y=w315:dbl[])
                      }
                      frame "pF".. {
                      }
                    }
                    n186 = local read "Initial volts [V]"() -> (w307:dbl)
                    n187 = Bundle("Initial volts [V]"=w307, w308, w300) -> (w305:cluster{"Initial volts [V]":dbl, dbl, dbl[]})  [unwired: 1 in]
                    n188 = local write "Cgraph"(w305) -> ()
                  }
                }
                n189 = case shown="True" w287 {
                  tunnel: w286 -> [_ w321]
                  frame False {
                  }
                  frame True {
                    n190 = case shown="\"Log - log\".." w321 {
                      tunnel: [w322 1 0 w327] -> w320
                      tunnel: [w322 0 1 w327] -> w319
                      frame .."Lin - Lin" {
                        w322 = 0
                      }
                      frame "Log - Lin" {
                      }
                      frame "Lin - Log" {
                      }
                      frame "Log - log".. {
                        w327 = 1
                      }
                    }
                    n191 = property on="Cgraph" class="WFGraph (strict)"("X Scale.Mapping Mode"=w320) -> ()  [unwired: 2 in, 2 out]
                    n192 = property on="Cgraph" class="WFGraph (strict)"("Y Scale.Mapping Mode"=w319, "YScale.Minimum"=w319) -> ()  [unwired: 2 in, 2 out]
                  }
                }
                n193 = Subtract(x=w290, y=w273) -> (x-y=w272:dbl)
                n194 = Not(x=w289) -> (.not. x?=w295:bool)
                n195 = Greater Than 0?(x=w272) -> (x > 0?=w274:bool)
                n196 = Format Into String(format string="%d", w272) -> (resulting string=w294:string)  [unwired: 2 in, 1 out]
                n197 = And(x=w274, y=w295) -> (x .and. y?=w292:bool)
                n198 = Concatenate Strings(w278, "\r\n", "Timer status: ", w294) -> (w288:string)
                n199 = local write "STATUS 1"(w288) -> ()
              }
            }
            frame #1 {
              n200 = local read "abort"() -> (w329:bool)
              n201 = case shown="False" w329 {
                tunnel: w330 -> [w336 _]
                tunnel: w331 -> [w335 _]
                tunnel: w332 -> [w334 _]
                tunnel: [w333 FALSE] -> w328
                frame False {
                  n202 = stacked-sequence {
                    seq-local: [w362 _] -> [_ w386]
                    seq-local: [w361 _] -> [_ _]
                    seq-local: [w348 _] -> [_ _]
                    tunnel: w334 -> [_ w398]
                    tunnel: w335 -> [_ _]
                    tunnel: w336 -> [_ _]
                    tunnel: [w364 _] -> w333
                    frame #0 {
                      w344 = T3."Write Element" ("Action")
                      # "SMU data"
                      n203 = Get Date/Time String(want seconds? (F)=TRUE) -> (time string=w363:string)  [unwired: 2 in, 1 out]
                      n204 = local write "Last reading at:"(w363) -> ()
                      n205 = local write "STATUS 1"("Reading LCR meter..." ("status")) -> ()
                      n206 = global read "QC_MeasurementSetup.vi" "Cis Measurement Parameters"() -> (w360:T8)
                      n207 = Unbundle By Name(w360) -> ("Temperature Readout"=w338:enum16{"Read Arduino", "Enter manually"}, "Arduino"=w337:refnum<class "ArduinoControl.lvclass">, "LCR"=w354:refnum<class "LCRControl.lvclass">, "AC frequency [Hz]"=w339:i32, "Supply"=w355:refnum<class "SupplyControl.lvclass">, "Set Current Limit?"=w359:bool, "Current Limit [µA]"=w357:dbl)
                      n208 = local read "Current reading No."() -> (w343:u32)
                      n209 = case shown="\"Read Arduino\"" w338 {
                        tunnel: [w371 w374] -> w341
                        tunnel: [w368 w377] -> w346
                        tunnel: w337 -> [_ w376]
                        frame "Enter manually", Default {
                          n210 = local read "Temp."() -> (w373:dbl[])
                          n211 = local read "RH"() -> (w369:dbl[])
                          n212 = Index Array(array=w373, index=0) -> (element=w371:dbl)
                          n213 = Index Array(array=w369, index=0) -> (element=w368:dbl)
                        }
                        frame "Read Arduino" {
                          n214 = call "ArduinoRead.vi"("Arduino function"=enum16{"T/RH", "Interlock", "Edgesense"}."T/RH", "ArduinoControl in"=w376) -> ("rel. Humidity [%]"=w377:dbl, "Temperature [°C]"=w374:dbl)  [unwired: 4 in, 4 out]
                        }
                      }
                      n215 = local read "Current Volts:"() -> (w347:dbl)
                      n216 = Multiply(x=w357, y=1000.0) -> (x*y=w356:dbl)
                      n217 = call-dynamic "Supply_ReadCurrent.vi"("SupplyControl in"=w355) -> ("error out"=w349:errorcluster, "Current in nA"=w365:dbl, "SupplyControl out"=w361:refnum<class "SupplyControl.lvclass">)  [unwired: 8 in]
                      n218 = case shown="True" w359 {
                        tunnel: w365 -> [_ w382]
                        tunnel: w356 -> [_ w380]
                        tunnel: [FALSE w379] -> w364
                        frame False {
                        }
                        frame True {
                          n219 = Absolute Value(x=w382) -> (abs(x)=w381:dbl)
                          n220 = Greater?(x=w381, y=w380) -> (0:w379:bool)
                        }
                      }
                      n221 = call "CisData.vi"("Action"=w344, "Array No."=0, "Array Size / Index"=w343, "Data IN"=w347) -> ()  [unwired: 1 in, 2 out]
                      n222 = call-dynamic "LCR_Readout.vi"("error in (no error)"=w349, "Frequency in Hz"=w339, "LCRControl in"=w354) -> ("error out"=w348:errorcluster, "Resistance in Ohm"=w342:dbl, "Capacitance in pF"=w340:dbl)  [unwired: 5 in, 1 out]
                      n223 = Increment(x=w343) -> (x+1=w362:u32)
                      n224 = local write "Current reading No."(w362) -> ()
                      n225 = call "CisData.vi"("Action"=w344, "Array No."=u32 1, "Array Size / Index"=w343, "Data IN"=w340) -> ()  [unwired: 1 in, 2 out]
                      n226 = call "CisData.vi"("Action"=w344, "Array No."=u32 2, "Array Size / Index"=w343, "Data IN"=w342) -> ()  [unwired: 1 in, 2 out]
                      n227 = call "CisData.vi"("Action"=w344, "Array No."=u32 3, "Array Size / Index"=w343, "Data IN"=w341) -> ()  [unwired: 1 in, 2 out]
                      n228 = call "CisData.vi"("Action"=w344, "Array No."=u32 4, "Array Size / Index"=w343, "Data IN"=w346) -> ()  [unwired: 1 in, 2 out]
                    }
                    frame #1 {
                      w395 = u32 5 ("y")
                      # "Update plots"
                      n229 = property on="Cgraph" class="WFGraph (strict)"() -> ("YScale.Mapping Mode"=w387:u8)  [unwired: 2 in, 2 out]
                      n230 = Greater?(x=w386, y=w395) -> (0:w394:bool)
                      n231 = call "CisData.vi"("Action"=T3."Read Array", "Array No."=1) -> ("Array OUT"=w384:dbl[])  [unwired: 3 in, 1 out]
                      n232 = case shown="True" w394 {
                        tunnel: w386 -> [w403 w406]
                        tunnel: w395 -> [_ w405]
                        tunnel: [w403 w405] -> w393
                        tunnel: [0 w404] -> w391
                        frame False {
                        }
                        frame True {
                          n233 = Subtract(x=w406, y=w405) -> (x-y=w404:u32)
                        }
                      }
                      n234 = property on="Cgraph" class="WFGraph (strict)"("YScale.Minimum"=w387) -> ()  [unwired: 2 in, 2 out]
                      n235 = Array Subset(array=w384, index=0, length=w386) -> (w390:dbl[])
                      n236 = local read "Cscale"() -> (w396:enum16{"1/C^2 [1/nF^2]", "nF", "pF"})
                      n237 = Absolute Value(x=w390) -> (abs(x)=w389:dbl[])
                      n238 = case shown="..\"1/C^2 [1/nF^2]\"" w396 {
                        tunnel: [w439 w442 w445] -> w401
                        tunnel: w389 -> [w437 w444 w445]
                        frame .."1/C^2 [1/nF^2]" {
                          n239 = Array Size(array=w437) -> (size(s)=w438:i32)
                          n240 = for {
                            N: w438 -> [_]
                            tunnel: w437 -> [w441] mode=indexing
                            tunnel: [w440] -> w439 mode=indexing
                            n241 = formula code="y=1000000./(x*x);"("x"=w441) -> ("y"=w440:dbl)
                          }
                        }
                        frame "nF" {
                          n242 = Divide(x=w444, y=1000.0) -> (x/y=w442:dbl[])
                        }
                        frame "pF".. {
                        }
                      }
                      n243 = for {
                        N: 5 -> [_]
                        tunnel: w393 -> [w412]
                        tunnel: w391 -> [w411]
                        tunnel: w386 -> [w410]
                        i -> [w408]
                        n244 = call "CisData.vi"("Action"=T3."Read Array", "Array No."=w408) -> ("Array OUT"=w407:dbl[])  [unwired: 3 in, 1 out]
                        n245 = case shown="2" w408 {
                          tunnel: w412 -> [w415 w419 w424 _ _]
                          tunnel: w411 -> [w416 w420 w425 _ _]
                          tunnel: w407 -> [w414 w418 w426 w430 w435]
                          tunnel: w410 -> [_ _ _ w428 w433]
                          frame ..0 {
                            n246 = Array Subset(array=w414, index=w416, length=w415) -> (w413:dbl[])
                            n247 = local write "Volts"(w413) -> ()
                          }
                          frame 1 {
                            n248 = Array Subset(array=w418, index=w420, length=w419) -> (w417:dbl[])
                            n249 = local write "Capacitance"(w417) -> ()
                          }
                          frame 2 {
                            n250 = Array Subset(array=w426, index=w425, length=w424) -> (w422:dbl[])
                            n251 = Multiply(x=w422, y=0.001) -> (x*y=w421:dbl[])
                            n252 = local write "Resistance"(w421) -> ()
                          }
                          frame 3 {
                            n253 = Decrement(x=w428) -> (x-1=w427:u32)
                            n254 = Array Subset(array=w430, index=w427, length=1) -> (w429:dbl[])
                            n255 = local write "Temp."(w429) -> ()
                          }
                          frame 4.. {
                            n256 = Decrement(x=w433) -> (x-1=w432:u32)
                            n257 = Array Subset(array=w435, index=w432, length=1) -> (w434:dbl[])
                            n258 = local write "RH"(w434) -> ()
                          }
                        }
                      }
                      n259 = local read "Initial volts [V]"() -> (w399:dbl)
                      n260 = Absolute Value(x=w398) -> (abs(x)=w397:dbl)
                      n261 = Bundle("Initial volts [V]"=w399, w397, w401) -> (w388:cluster{"Initial volts [V]":dbl, dbl, dbl[]})  [unwired: 1 in]
                      n262 = local write "Cgraph"(w388) -> ()
                    }
                  }
                }
                frame True {
                }
              }
            }
          }
          n263 = Build Array("abort", w254) -> (w260:bool[])
        }
        frame True {
          w447 = FALSE
          # "compliance was exceeded when first voltage applied."
          # "Flag compliance as reason for end of run"
          n264 = local write "STATUS 1"("Run aborted - compliance exceeded.") -> ()
          n265 = Build Array(w447, TRUE, w447, w447) -> (w448:bool[])
        }
      }
      n266 = Search 1D Array(1D array=w246, element=TRUE) -> (index of element=w244:i32)  [unwired: 1 in]
      n267 = Increment(x=w244) -> (x+1=w243:i32)
      n268 = case shown="..0" w243 {
        tunnel: ["" "Run ended normally" "Compliance exceeded" "Run aborted - by user" "Run aborted - Ilimit exceeded"] -> w238
        frame ..0 {
        }
        frame 1 {
        }
        frame 2 {
          # "Determine reason for end of run."
        }
        frame 3 {
        }
        frame 4.. {
        }
      }
      n269 = global read "QC_RunInformation.vi" "Run info"() -> (w242:T6)
      n270 = Bundle By Name(cluster=w242, "End of Run comment:"=w238) -> (w237:T6)
      n271 = Concatenate Strings(w238, "\r\n", "RAMPING DOWN VOLTS") -> (w241:string)
      n272 = global write "QC_RunInformation.vi" "Run info"(w237) -> ()
      n273 = local write "STATUS 1"(w241) -> ()
    }
    frame #4 {
      # "Ramp down and switch off supply"
      n274 = stacked-sequence {
        frame #0 {
          # "Tie up loose ends. Set volts to zero and switch to standby"
          # "Ramp down volts now"
          n275 = global read "QC_MeasurementSetup.vi" "Cis Measurement Parameters"() -> (w459:T8)
          n276 = Unbundle By Name(w459) -> ("Supply"=w456:refnum<class "SupplyControl.lvclass">, "Ramp down steps [V]"=w458:dbl, "Ramp down Interval [s]"=w457:i32, "Switching"=w452:refnum<class "Switching.lvclass">, "Matrix used?"=w453:bool)
          n277 = local read "Current Volts:"() -> (w464:dbl)
          n278 = Multiply(x=w457, y=1000) -> (x*y=w461:i32)
          n279 = call "SupplyRamp.vi"("Requested Voltage"=0.0, "Step Size"=w458, "Step Delay"=w461, "Supply IN"=w456, "Starting Voltage"=w464) -> ("error out"=w455:errorcluster, "Supply OUT"=w454:refnum<class "SupplyControl.lvclass">, "Current Voltage"=w462:dbl)  [unwired: 3 in, 1 out]
          n280 = call-dynamic "Supply_Stby.vi"("error in (no error)"=w455, "SupplyControl in"=w454) -> ("error out"=w451:errorcluster)  [unwired: 8 in, 1 out]
          n281 = local write "Current Volts:"(w462) -> ()
          n282 = case shown="True" w453 {
            tunnel: w452 -> [_ w469]
            tunnel: w451 -> [_ w468]
            frame False {
            }
            frame True {
              n283 = call-dynamic "MatrixSwitch.vi"("error in (no error)"=w468, "Action"=T4."Reset", "Switching in"=w469) -> ("error out"=w465:errorcluster, "Switching out"=w466:refnum<class "Switching.lvclass">)  [unwired: 6 in, 1 out]
              n284 = call-dynamic "Close.vi"("error in (no error)"=w465, "Switching in"=w466) -> ()  [unwired: 8 in, 2 out]
            }
          }
        }
        frame #1 {
          w474 = 0
          n285 = local write "Bias On/Off:"(FALSE ("Visible")) -> ()
          n286 = local write "Current Volts:"(0.0 ("Current Volts:")) -> ()
          n287 = property on="abort" class="Bool (strict)"("DisabledEnum"=2) -> ()  [unwired: 2 in, 2 out]
          n288 = property on="Quit & Save" class="Bool"("DisabledEnum"=w474) -> ()  [unwired: 2 in, 2 out]
          n289 = property on="quit (no save)" class="Bool"("DisabledEnum"=w474) -> ()  [unwired: 2 in, 2 out]
          n290 = local write "STATUS 1"("Run finished. \nSave data?" ("STATUS 1")) -> ()
        }
        frame #2 {
          n291 = Current VI's Path() -> (path=w476:path)
          n292 = call "SaveJPEG.vi"("Test"="Cis", "File Path Control"=w476) -> ()  [unwired: 1 in, 2 out]
        }
      }
    }
    frame #5 {
      # "Loop and await decision on whether to save or junk data"
      # "Display and save data"
      n293 = local read "Cscale"() -> (w486:enum16{"1/C^2 [1/nF^2]", "nF", "pF"})
      n294 = local read "Scales"() -> (w487:T1)
      n295 = while {
        shift-left: w486 -> [w534]
        shift-right: [w533] -> _
        shift-left: w487 -> [w536]
        shift-right: [w535] -> _
        tunnel: ["Quit & Save"] -> w489
        tunnel: ["quit (no save)"] -> w488
        stop <- w531 continue-if-true
        n296 = local read "Scales"() -> (w535:T1)
        n297 = local read "Cscale"() -> (w533:enum16{"1/C^2 [1/nF^2]", "nF", "pF"})
        n298 = Not Equal?(x=w536, y=w535) -> (x != y?=w529:bool)
        n299 = Not Equal?(x=w534, y=w533) -> (x != y?=w528:bool)
        n300 = case shown="True" w529 {
          tunnel: w535 -> [_ w563]
          frame False {
          }
          frame True {
            n301 = case shown="\"Log - log\".." w563 {
              tunnel: [w564 1 0 w569] -> w562
              tunnel: [w564 0 1 w569] -> w561
              frame .."Lin - Lin" {
                w564 = 0
              }
              frame "Log - Lin" {
              }
              frame "Lin - Log" {
              }
              frame "Log - log".. {
                w569 = 1
              }
            }
            n302 = property on="Cgraph" class="WFGraph (strict)"("X Scale.Mapping Mode"=w562) -> ()  [unwired: 2 in, 2 out]
            n303 = property on="Cgraph" class="WFGraph (strict)"("Y Scale.Mapping Mode"=w561, "YScale.Minimum"=w561) -> ()  [unwired: 2 in, 2 out]
          }
        }
        n304 = case shown="True" w528 {
          tunnel: w533 -> [_ w541]
          frame False {
          }
          frame True {
            n305 = property on="Cgraph" class="WFGraph (strict)"() -> ("YScale.Mapping Mode"=w544:u8)  [unwired: 2 in, 2 out]
            n306 = global read "QC_MeasurementSetup.vi" "Cis Measurement Parameters"() -> (w543:T8)
            n307 = property on="Cgraph" class="WFGraph (strict)"("YScale.Minimum"=w544) -> ()  [unwired: 2 in, 2 out]
            n308 = Unbundle By Name(w543) -> ("Initial Voltage [V]"=w546:dbl, "Step Size [V]"=w548:dbl, "Number Of Steps"=w545:u32)
            n309 = call "CisData.vi"("Action"=T3."Read Array", "Array No."=u32 1 ("Action")) -> ("Array OUT"=w537:dbl[])  [unwired: 3 in, 1 out]
            n310 = Absolute Value(x=w548) -> (abs(x)=w547:dbl)
            n311 = Array Subset(array=w537, index=0, length=w545) -> (w549:dbl[])
            n312 = Absolute Value(x=w549) -> (abs(x)=w542:dbl[])
            n313 = case shown="..\"1/C^2 [1/nF^2]\"" w541 {
              tunnel: [w554 w557 w560] -> w540
              tunnel: w542 -> [w552 w559 w560]
              frame .."1/C^2 [1/nF^2]" {
                n314 = Array Size(array=w552) -> (size(s)=w553:i32)
                n315 = for {
                  N: w553 -> [_]
                  tunnel: w552 -> [w556] mode=indexing
                  tunnel: [w555] -> w554 mode=indexing
                  n316 = formula code="y=1000000./(x*x);"("x"=w556) -> ("y"=w555:dbl)
                }
              }
              frame "nF" {
                n317 = Divide(x=w559, y=1000.0) -> (x/y=w557:dbl[])
              }
              frame "pF".. {
              }
            }
            n318 = Bundle("Initial Voltage [V]"=w546, w547, w540) -> (w550:cluster{"Initial Voltage [V]":dbl, dbl, dbl[]})  [unwired: 1 in]
            n319 = local write "Cgraph"(w550) -> ()
          }
        }
        n320 = Not Or(1:"quit (no save)", 2:"Quit & Save") -> (0:w531:bool)
      }
      n321 = global read "QC_MeasurementSetup.vi" "Cis Measurement Parameters"() -> (w485:T8)
      n322 = Unbundle By Name(w485) -> ("Temperature Readout"=w484:enum16{"Read Arduino", "Enter manually"}, "Arduino"=w478:refnum<class "ArduinoControl.lvclass">)
      n323 = case shown="\"Read Arduino\"" w484 {
        tunnel: w478 -> [_ w527]
        frame "Enter manually", Default {
        }
        frame "Read Arduino" {
          n324 = call "ArduinoClose.vi"("ArduinoControl in"=w527) -> ()  [unwired: 9 in, 2 out]
        }
      }
      n325 = case shown="True" w488 {
        tunnel: [FALSE w571] -> w490
        frame False {
        }
        frame True {
          n326 = Two Button Dialog(message="Are you sure you don't want to save the data?", 1:"Quit" ("F button name (\"Cancel\")"), 2:"Save data" ("T button name (\"OK\")")) -> (T button?=w571:bool)
        }
      }
      n327 = Or(x=w489, y=w490) -> (x .or. y?=w483:bool)
      n328 = flat-sequence {
        tunnel: w483 -> [w492]
        tunnel: [w492] -> w479
        tunnel: [TRUE] -> w477
        frame #0 {
          n329 = global read "QC_MeasurementSetup.vi" "Cis Measurement Parameters"() -> (w502:T8)
          n330 = Unbundle By Name(w502) -> ("C_is Limit [pF/cm]"=w495:dbl, "Number Of Steps"=w497:u32)
          n331 = call "ScanFeedback.vi"("measurement type"=T5."Cis") -> ("Cis @300V [pF/cm]"=w493:dbl)  [unwired: 4 in, 4 out]
          n332 = case shown="True" w492 {
            tunnel: ["" w526] -> w503
            tunnel: [_ w511] -> w501
            tunnel: w497 -> [_ _]
            frame False {
            }
            frame True {
              w509 = T3."Read Array" ("Action")
              n333 = local write "STATUS 1"("Saving Data ...") -> ()
              n334 = call "CisData.vi"("Action"=w509, "Array No."=u32 2 ("Action")) -> ("Array OUT"=w507:dbl[])  [unwired: 3 in, 1 out]
              n335 = Multiply(x=w507, y=0.001) -> (x*y=w506:dbl[])
              n336 = call "CisData.vi"("Action"=w509, "Array No."=u32 0 ("Action")) -> ("Array OUT"=w517:dbl[])  [unwired: 3 in, 1 out]
              n337 = call "CisData.vi"("Action"=w509, "Array No."=u32 1 ("Action")) -> ("Array OUT"=w516:dbl[])  [unwired: 3 in, 1 out]
              n338 = Build Array(w517, w516, w506) -> (w515:dbl[][])
              n339 = call "CisData.vi"("Action"=w509, "Array No."=u32 4 ("Action")) -> ("Array OUT"=w523:dbl[])  [unwired: 3 in, 1 out]
              n340 = call "CisData.vi"("Action"=w509, "Array No."=u32 3 ("Action")) -> ("Array OUT"=w522:dbl[])  [unwired: 3 in, 1 out]
              n341 = call <vilib>:"Std Deviation and Variance.vi"("X"=w523) -> ("mean"=w512:dbl)  [unwired: 1 in, 2 out]
              n342 = call <vilib>:"Std Deviation and Variance.vi"("X"=w522) -> ("mean"=w513:dbl)  [unwired: 1 in, 2 out]
              n343 = Transpose 2D Array(2D array=w515) -> (transposed array=w514:dbl[][])
              n344 = call "SaveDataFile.vi"("Data Array"=w514, "Temperature"=w513, "Humidity"=w512, "Array Titles"="Voltage[V] Capacitance[pF] Resistance[kOhm]", "Strip Segment"="") -> ("Path + Filename OUT"=w526:string, "Error Out"=w511:errorcluster)  [unwired: 7 in, 2 out]
            }
          }
          n345 = Absolute Value(x=w493) -> (abs(x)=w496:dbl)
          n346 = Absolute Value(x=w495) -> (abs(x)=w494:dbl)
          n347 = Less Or Equal?(x=w496, y=w494) -> (x <= y?=w498:bool)
          n348 = call "WriteLogFile.vi"("Automatic warning"="", "Data File"=w503, "Error In"=w501, "DUT passed?"=w498, "Value TechSpec criteria"=w493, "Files saved?"=w492) -> ()  [unwired: 5 in, 1 out]
        }
      }
      n349 = Select(t="Run finished.\nData saved." ("STATUS 1"), s=w479, f="Run finished.\nData not saved." ("STATUS 1")) -> (s? t:f=w482:string)
      n350 = local write "STATUS 1"(w482) -> ()
      "Done!" <- w477
    }
  }
